vi "全局 时间.vi"() -> ()   [LabVIEW 2016]
panel:
  in  "时间":string
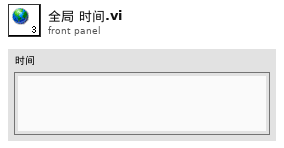
[diagram p1: front panel]
diagram:
